vi "Main.vi"() -> ()   [LabVIEW 2021]
doc: "The myRIO Project template acquires acceleration data from the onboard accelerometer and displays the changes of acceleration values in a waveform chart."
uses:
  <vilib>/myRIO/Instrument Drivers/Onboard IO/I2C/typedefs/I2C User Configuration.ctl
  <vilib>/myRIO/Instrument Drivers/Onboard IO/I2C/typedefs/I2C Transfer Rate.ctl
  <vilib>/myRIO/Instrument Drivers/Onboard IO/DIO/typedefs/DIO Reference.ctl
  <vilib>/myRIO/Common/Instrument Driver Framework/Utilities/typedefs/myRIO Generic Hardware Reference.ctl
  <vilib>/myRIO/Common/Instrument Driver Framework/Utilities/typedefs/Hardware Version Enum.ctl
  <vilib>/myRIO/Common/Instrument Driver Framework/Utilities/typedefs/myRIO v1.0 Reference.ctl
  <vilib>/myRIO/Common/Instrument Driver Framework/Utilities/typedefs/Generic FPGA Reference.ctl
  <vilib>/myRIO/Common/Instrument Driver Framework/myRIO v1.0/DIO/typedefs/DIO Channels List.ctl
  <vilib>/myRIO/Common/Instrument Driver Framework/myRIO v1.0/DIO/typedefs/DIO Channels Enum.ctl
  <vilib>/userDefined/High Color/nirio_resource_hc.ctl
  <vilib>/myRIO/Instrument Drivers/Onboard IO/I2C/typedefs/I2C Reference.ctl
  <vilib>/myRIO/Common/Instrument Driver Framework/myRIO v1.0/I2C/typedefs/I2C Channels Enum.ctl
  <vilib>/myRIO/Instrument Drivers/Onboard IO/I2C/typedefs/I2C Configuration.ctl
  <vilib>/Platform/TimedLoop/XDataNode/timing_clust.ctl
  <vilib>/Platform/TimedLoop/XDataNode/nitl_modes.ctl
  <vilib>/Platform/TimedLoop/XDataNode/wakeup.ctl
  sketch_state.ctl
  <vilib>/myRIO/Instrument Drivers/Onboard IO/UART/typedef/VISA Configuration.ctl
  <vilib>/myRIO/Instrument Drivers/Onboard IO/SPI/typedefs/SPI User Configuration.ctl
  <vilib>/myRIO/Common/Instrument Driver Framework/myRIO v1.0/SPI/typedefs/SPI Clock Phase.ctl
  <vilib>/myRIO/Common/Instrument Driver Framework/myRIO v1.0/SPI/typedefs/SPI Clock Polarity.ctl
  <vilib>/myRIO/Common/Instrument Driver Framework/myRIO v1.0/SPI/typedefs/SPI Data Direction.ctl
  <vilib>/myRIO/Common/Instrument Driver Framework/myRIO v1.0/SPI/typedefs/SPI Frame Length.ctl
  <vilib>/myRIO/Instrument Drivers/Onboard IO/SPI/typedefs/SPI Reference.ctl
  <vilib>/myRIO/Common/Instrument Driver Framework/myRIO v1.0/SPI/typedefs/SPI Channels Enum.ctl
  <vilib>/myRIO/Instrument Drivers/Onboard IO/SPI/typedefs/SPI Configuration.ctl
  <vilib>/myRIO/Common/Instrument Driver Framework/myRIO v1.0/DIO/vis/myRIO v1.1 Open DIO.vi
  <vilib>/myRIO/Common/Instrument Driver Framework/myRIO v1.0/I2C/vis/myRIO v1.1 Open I2C.vi
  <vilib>/myRIO/Common/Instrument Driver Framework/Utilities/vis/Is FPGA Ref Available.vi
  <vilib>/myRIO/Common/Instrument Driver Framework/myRIO v1.0/SPI/vis/myRIO v1.1 Open SPI.vi
  <vilib>/myRIO/Common/Instrument Driver Framework/Utilities/vis/Validate Channels.vi
  <vilib>/myRIO/Common/Instrument Driver Framework/myRIO v1.0/DIO/vis/myRIO v1.0 Reserve DIO.vi
  <vilib>/myRIO/Common/Instrument Driver Framework/myRIO v1.0/I2C/vis/myRIO v1.0 Reserve I2C.vi
  <vilib>/myRIO/Common/Instrument Driver Framework/myRIO v1.0/SPI/vis/myRIO v1.0 Reserve SPI.vi
  <vilib>/myRIO/Common/Instrument Driver Framework/myRIO v1.0/DIO/vis/myRIO v1.0 Close DIO.vi
  <vilib>/myRIO/Common/Instrument Driver Framework/myRIO v1.0/Resource Manager/vis/myRIO v1.0 Reserve Channel List.vi
  <vilib>/myRIO/Common/Instrument Driver Framework/myRIO v1.0/DIO/vis/myRIO v1.0 Build MUX Configuration DIO.vi
  <vilib>/myRIO/Common/Instrument Driver Framework/myRIO v1.0/I2C/vis/myRIO v1.0 Build MUX Configuration I2C.vi
  <vilib>/myRIO/Common/Instrument Driver Framework/myRIO v1.0/SPI/vis/myRIO v1.0 Build MUX Configuration SPI.vi
  <vilib>/myRIO/Common/Instrument Driver Framework/myRIO v1.0/DIO/vis/myRIO v1.0 Unreserve DIO.vi
  <vilib>/myRIO/Common/Instrument Driver Framework/myRIO v1.0/Resource Manager/vis/myRIO v1.0 Reserve Channel.vi
  <vilib>/myRIO/Common/Instrument Driver Framework/myRIO v1.0/Resource Manager/vis/myRIO v1.0 Unreserve Channel.vi
  <vilib>/myRIO/Common/Instrument Driver Framework/myRIO v1.0/Resource Manager/vis/myRIO v1.0 Create Configuration List.vi
  <vilib>/myRIO/Common/Instrument Driver Framework/myRIO v1.0/Resource Manager/vis/myRIO v1.0 Unreserve Channel List.vi
  <vilib>/myRIO/Common/Instrument Driver Framework/myRIO v1.0/Resource Manager/vis/myRIO v1.0 Build Mutex Name.vi
  <vilib>/Utility/VariantDataType/GetNumericInfo.vi
  <vilib>/Utility/error.llb/Error Cluster From Error Code.vi
  <vilib>/myRIO/Common/Instrument Driver Framework/myRIO v1.0/myRIO v1.1 Open.vi
  <vilib>/myRIO/Common/Instrument Driver Framework/Utilities/vis/IO Manager.vi
  <vilib>/myRIO/Common/Instrument Driver Framework/Utilities/vis/Configuration Manager.vi
  <vilib>/myRIO/Common/Instrument Driver Framework/myRIO v1.0/Resource Manager/vis/myRIO v1.0 Configure IO.vi
  <vilib>/myRIO/Common/Instrument Driver Framework/myRIO v1.0/myRIO v1.0 Close.vi
  <vilib>/myRIO/Common/Instrument Driver Framework/myRIO v1.0/I2C/vis/myRIO v1.0 Configure I2C.vi
  <vilib>/myRIO/Common/Instrument Driver Framework/myRIO v1.0/I2C/vis/myRIO v1.0 Write I2C.vi
  <vilib>/Instr/_visa.llb/VISA Configure Serial Port (Instr).vi
  <vilib>/myRIO/Common/Instrument Driver Framework/myRIO v1.0/DIO/vis/myRIO v1.0 Write DIO.vi
  <vilib>/myRIO/Common/Instrument Driver Framework/myRIO v1.0/SPI/vis/myRIO v1.0 Configure SPI.vi
  <vilib>/myRIO/Common/Instrument Driver Framework/myRIO v1.0/SPI/vis/myRIO v1.0 Write Read SPI.vi
  <vilib>/myRIO/Common/Instrument Driver Framework/myRIO v1.0/DIO/vis/myRIO v1.0 Read DIO.vi
  <vilib>/myRIO/Common/Instrument Driver Framework/myRIO v1.0/I2C/vis/myRIO v1.0 Read I2C.vi
  <vilib>/myRIO/Common/Instrument Driver Framework/myRIO v1.0/DIO/vis/myRIO v1.0 Shutdown DIO.vi
  <vilib>/myRIO/Instrument Drivers/Onboard IO/DIO/vis/myRIO DIO Open.xnode
  <vilib>/myRIO/Instrument Drivers/Onboard IO/I2C/vis/myRIO I2C Open.xnode
  <vilib>/platform/TimedLoop/XDataNode/XDataNode.xnode
  <vilib>/myRIO/Express VI/Onboard IO/UART/UART Express VI.xnode
  <vilib>/myRIO/Express VI/Onboard IO/DO/DO Express VI.xnode
  <vilib>/myRIO/Express VI/Onboard IO/SPI/SPI Express VI.xnode
  <vilib>/myRIO/Instrument Drivers/Onboard IO/SPI/vis/myRIO SPI Open.xnode
  <vilib>/Platform/TimedLoop/XDataNode/XDNodeRunTimeDep.lvlib
  <vilib>/myRIO/Instrument Drivers/Onboard IO/DIO/DIO.lvlib
  <vilib>/myRIO/Instrument Drivers/Onboard IO/I2C/I2C.lvlib
  <vilib>/myRIO/Instrument Drivers/Onboard IO/SPI/SPI.lvlib
  <vilib>/myRIO/Instrument Drivers/Onboard IO/UART/UART.lvlib
panel:
  out "Bytes Read":u8[](array[numeric]) format="%x"
  out "X":i16
  out "Y":i16
  out "Z":i16
  in  "Stop Button":bool
  out "Waveform Chart":cluster{i16, i16, i16}(graph)
  out "INT_Source":bool[](array[boolean])
  out "Distance to Cabin":dbl
  out "Map":picture
  in  "Reset":bool
  in  "Left 2":bool
  in  "Forward":bool
  in  "Right 2":bool
  in  "Back":bool
  out "Light Detection":u8[](array[knob]) scale=0.0..255.0
  in  "Tree  Warning Dist (<)":u32
  out "Tree Warning":bool
  out "Ambient Temperature":dbl(slide) scale=0.0..40.0
  out "Alert":bool
  out "Ta":u8[](array[numeric])
  out "Thyst (hysteresis)":u8[](array[numeric]) format="%x"
  out "TSet":u8[](array[numeric]) format="%x"
  out "Sonic Distance (in)":u32
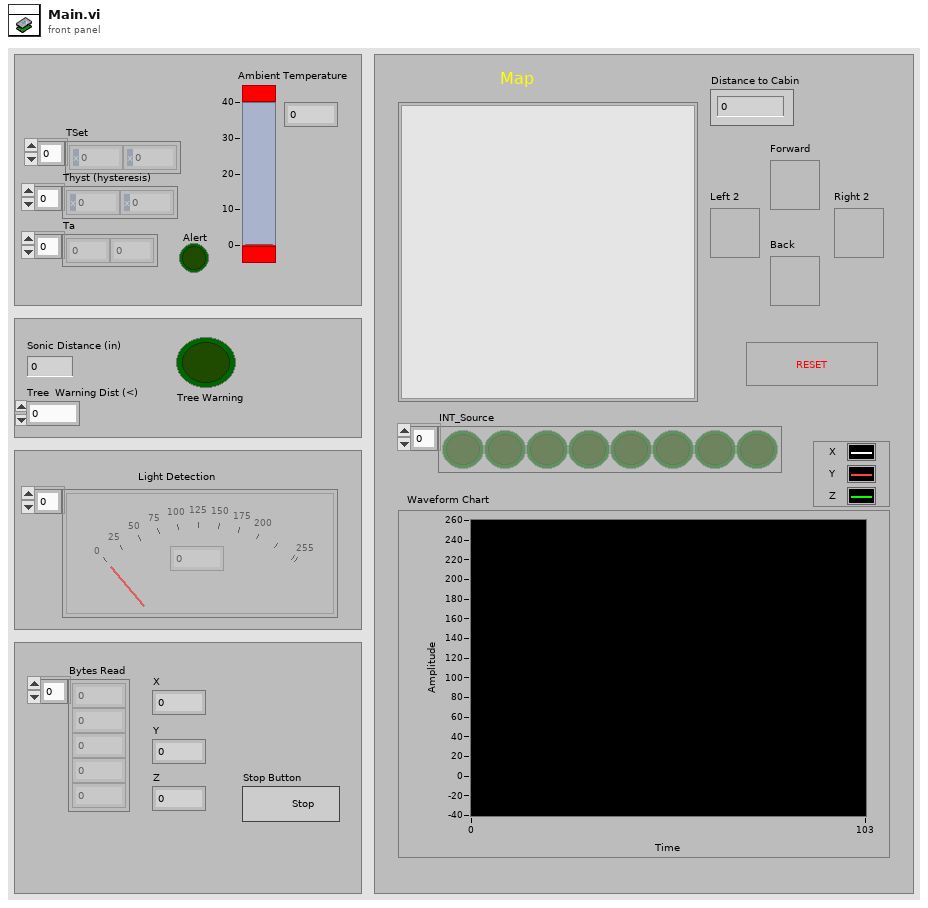
[diagram p1: front panel]
types:
  T1 = typedef "nirio_resource_hc.ctl" = tag
  T2 = typedef "Hardware Version Enum.ctl" = enum16{"Unknown", "myRIO-1900", "myRIO-1950", "roboRIO", "NI ELVIS RIO CM", "ELVIS III"}
  T3 = typedef "sketch_state.ctl" = enum16{"erase", "wait", "write"}
  T4 = typedef "UART.lvlib/VISA Configuration.ctl" = cluster{"baud rate (9600)":u32, "data bits (8)":u16, "parity (0:none)":enum16{"None", "Odd", "Even", "Mark", "Space"}, "stop bits (10: 1 bit)":u16, "flow control (0:none)":u16, "termination char\n(0xA = '\\n' = LF) ":u8, "Enable Termination\nChar (T)":bool, "timeout (10sec)":u32}
  T5 = typedef "DIO.lvlib/DIO Reference.ctl" = cluster{"myRIO Reference":T6, "DIO Channels List":T9}
  T6 = typedef "myRIO Generic Hardware Reference.ctl" = cluster{"myRIO Model":T2, "myRIO Hardware Reference":T7}
  T7 = typedef "myRIO v1.0 Reference.ctl" = cluster{"Generic FPGA Reference":T8, "Allow multiple opens":bool}
  T8 = typedef "Generic FPGA Reference.ctl" = refnum<k20>
  T9 = typedef "DIO Channels List.ctl" = T10[]
  T10 = typedef "DIO Channels Enum.ctl" = enum16{"Not Connected", "C/DIO0", "C/DIO1", "C/DIO2", "C/DIO3", "C/DIO4", "C/DIO5", "C/DIO6", "C/DIO7", "A/DIO0", "A/DIO1", "A/DIO2", "A/DIO3", "A/DIO4", "A/DIO5", "A/DIO6", "A/DIO7", "A/DIO8", "A/DIO9", "A/DIO10", "A/DIO11", "A/DIO12", "A/DIO13", "A/DIO14", "A/DIO15", "A/DIO16", "A/DIO17", "A/DIO18", "A/DIO19", "B/DIO0", "B/DIO1", "B/DIO2", "B/DIO3", "B/DIO4", "B/DIO5", "B/DIO6", "B/DIO7", "B/DIO8", "B/DIO9", "B/DIO10", "B/DIO11", "B/DIO12", "B/DIO13", "B/DIO14", "B/DIO15", "B/DIO16", "B/DIO17", "B/DIO18", "B/DIO19", "LED0", "LED1", "LED2", "LED3", "Button0", "DIO/DIO0", "DIO/DIO1", "DIO/DIO2", "DIO/DIO3", "DIO/DIO4", "DIO/DIO5", "DIO/DIO6", "DIO/DIO7", "DIO/DIO8", "DIO/DIO9", "SPI/CS0", "SPI/CS1", "SPI/CS2", "SPI/CS3", "LED RADIO (Green)", "LED RADIO (Red)", "LED COMM (Green)", "LED COMM (Red)", "LED MODE (Green)", "LED MODE (Red)"}
  T11 = typedef "SPI.lvlib/SPI Reference.ctl" = cluster{"myRIO Reference":T6, "SPI Channels Enum":T12, "SPI Configuration":T13}
  T12 = typedef "SPI Channels Enum.ctl" = enum16{"Not Connected", "A/SPI", "B/SPI", "SPI/SPI"}
  T13 = typedef "SPI.lvlib/SPI Configuration.ctl" = cluster{"Frequency [Hz]":dbl, "Clock Phase":T14, "Clock Polarity":T15, "Data Direction":T16, "Frame Length":T17}
  T14 = typedef "SPI Clock Phase.ctl" = enum8{"Leading", "Trailing"}
  T15 = typedef "SPI Clock Polarity.ctl" = enum8{"Low", "High"}
  T16 = typedef "SPI Data Direction.ctl" = enum8{"Most significant bit first", "Least significant bit first"}
  T17 = typedef "SPI Frame Length.ctl" = u8
  T18 = typedef "SPI.lvlib/SPI User Configuration.ctl" = cluster{"Frequency [Hz]":dbl, "Clock Phase":T14, "Clock Polarity":T15, "Data Direction":T16, "Frame Length":T17}
  T19 = typedef "XDNodeRunTimeDep.lvlib/timing_clust.ctl" = cluster{"Expected End [f-1]":u64, "Actual End [f-1]":u64, "Finished Late? [f-1]":bool, "Expected End [i-1]":u64, "Actual End [i-1]":u64, "Finished Late? [i-1]":bool, "Expected Start [i]":u64, "Actual Start [i]":u64, "Expected Start [f]":u64, "Actual Start [f]":u64, "Source Name":string, "Structure Name":string, "Period":i64, "Deadline":i64, "Offset":i64, "Start":i64, "Priority":i32, "Timeout":i32, "Mode":T20, "Wakeup Reason":T21, "Error":errorcluster, "Source Type":string, "Secondary Source Type":string, "Global End Time":u64, "Global Start Time":u64, "Frame Duration":u64, "Iteration Duration":u64, "Assigned CPU":i32, "I/O Scan Engine Mode":u32}
  T20 = typedef "XDNodeRunTimeDep.lvlib/nitl_modes.ctl" = enum32{"No Change", "Process missed periods, maintain original phase", "Discard missed periods, maintain original phase", "Process missed periods, ignore original phase", "Discard missed periods, ignore original phase"}
  T21 = typedef "XDNodeRunTimeDep.lvlib/wakeup.ctl" = enum32{"Normal", "Aborted", "Asynchronous wakeup", "Timing source error", "Timed loop error", "Timeout"}
  T22 = typedef "I2C.lvlib/I2C User Configuration.ctl" = cluster{"I2C Transfer Rate":T23}
  T23 = typedef "I2C.lvlib/I2C Transfer Rate.ctl" = enum16{"Standard mode (100 kbps)", "Fast mode (400 kbps)"}
  T24 = typedef "I2C.lvlib/I2C Reference.ctl" = cluster{"myRIO Reference":T6, "I2C Channels Enum":T25, "I2C Configuration":T26}
  T25 = typedef "I2C Channels Enum.ctl" = enum16{"Not Connected", "A/I2C", "B/I2C", "I2C/I2C"}
  T26 = typedef "I2C.lvlib/I2C Configuration.ctl" = cluster{"I2C Transfer Rate":T23}
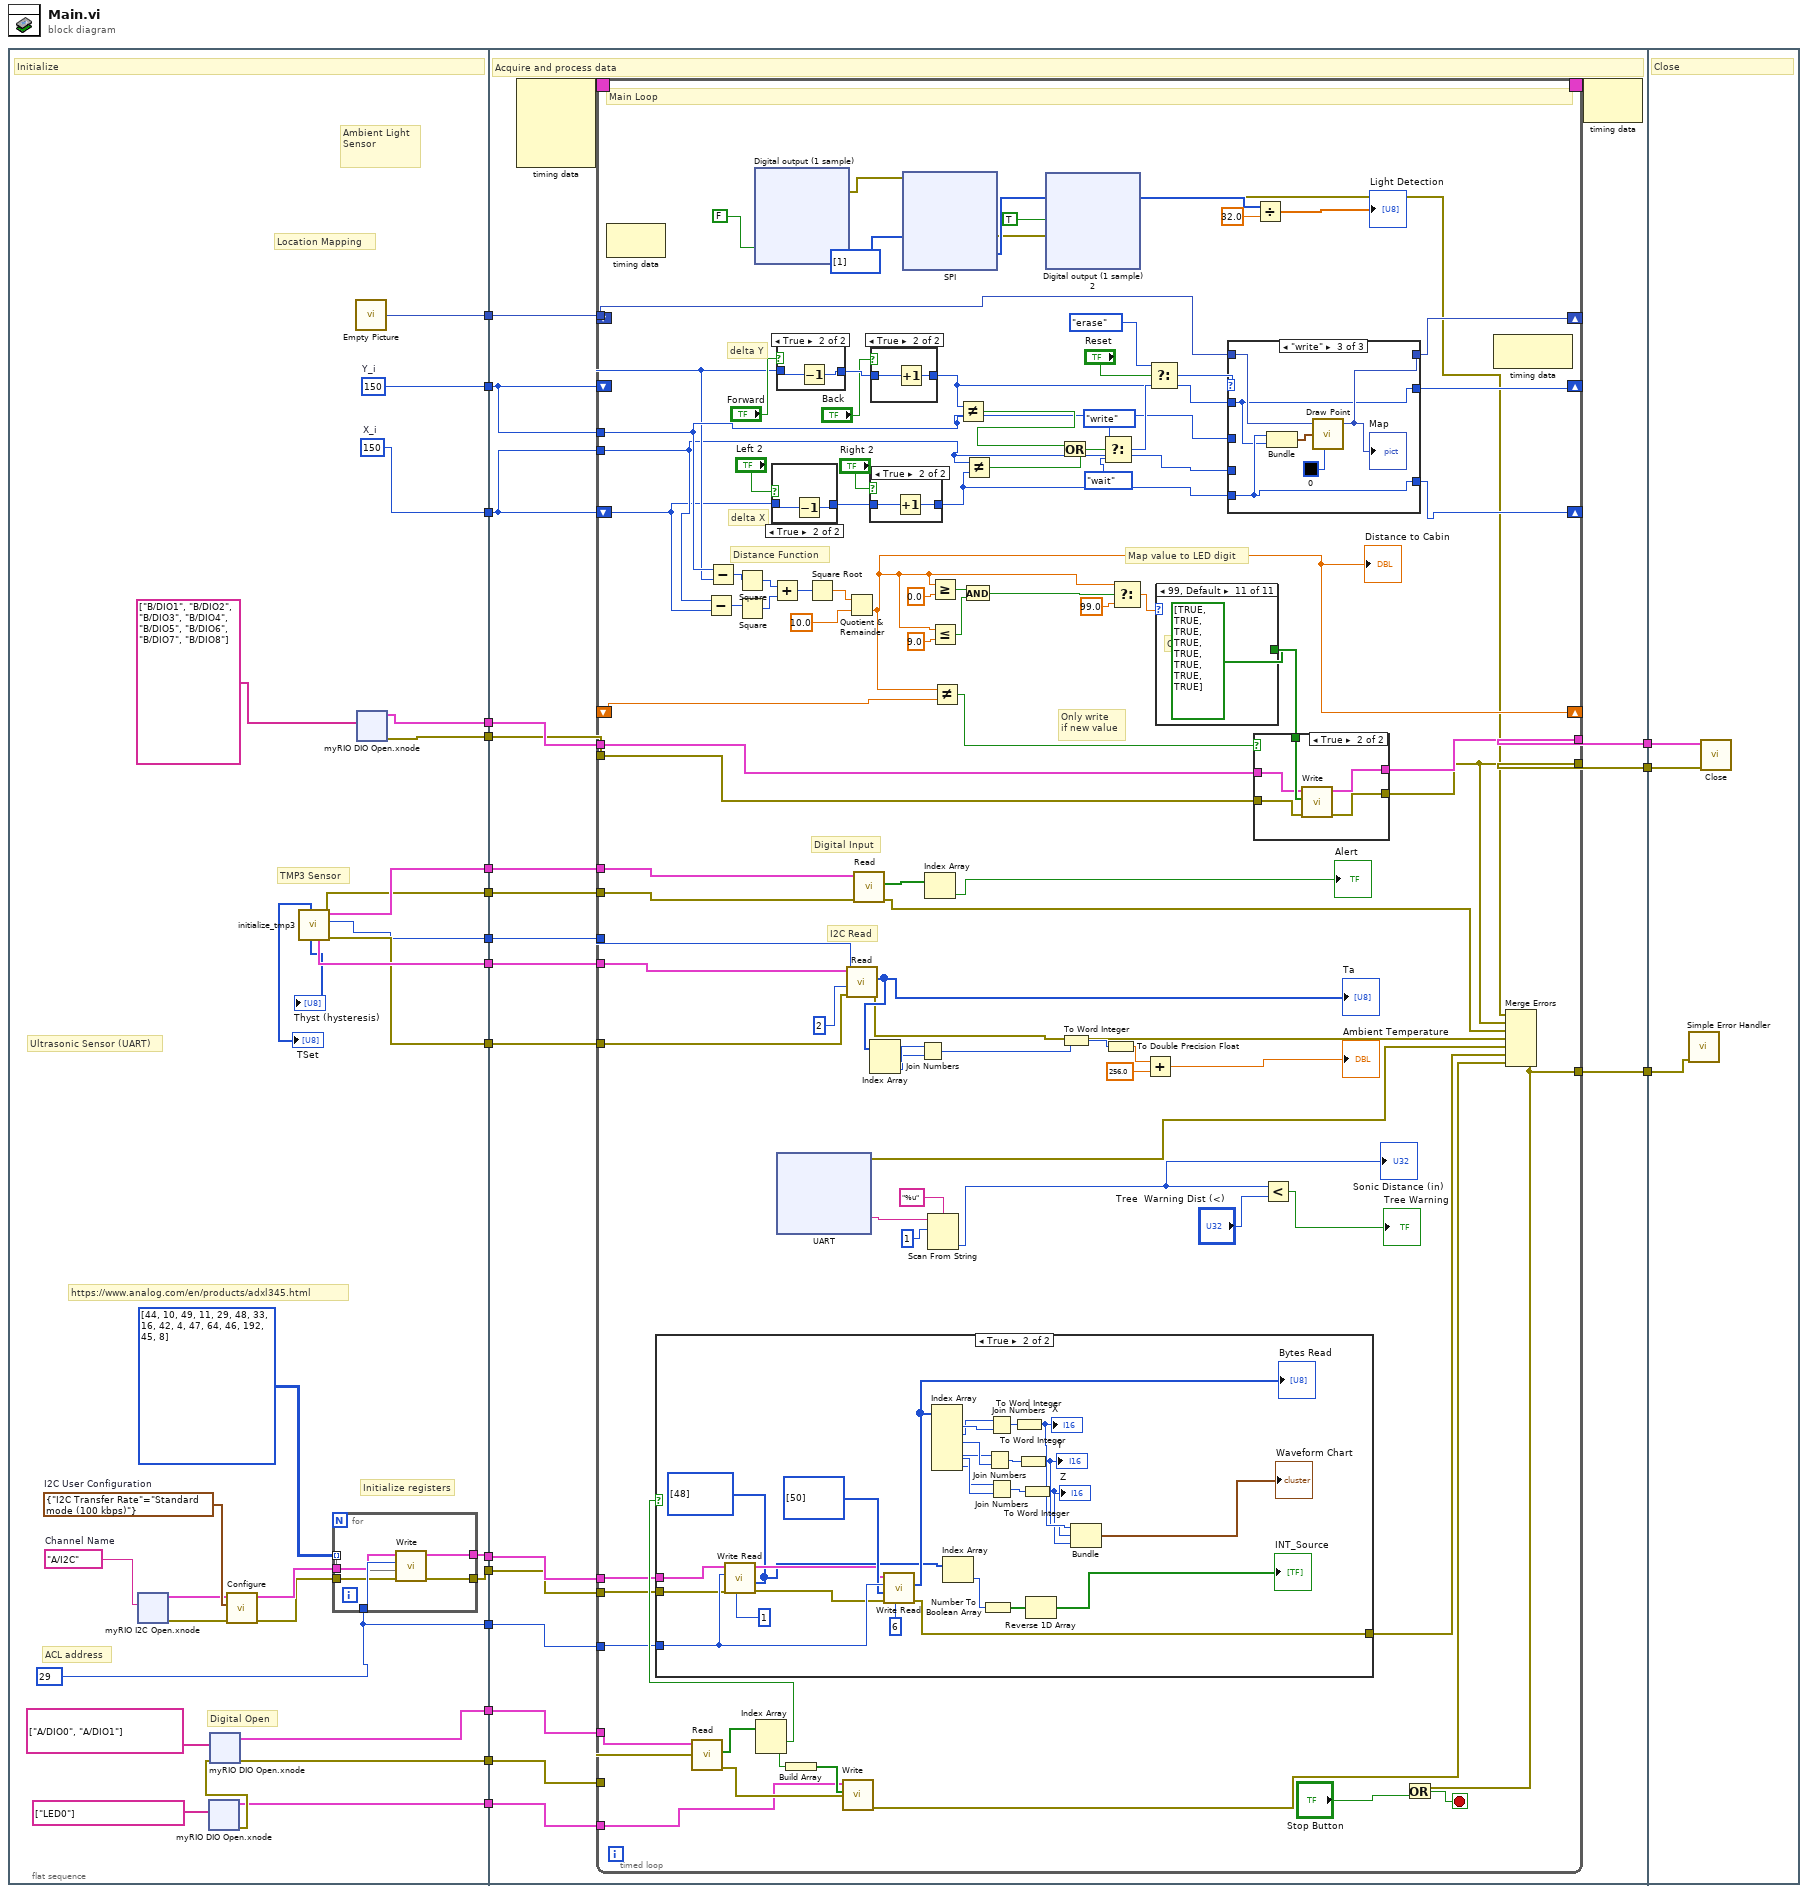
[diagram p0: block diagram]
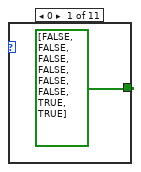
[diagram p4: hidden frame]
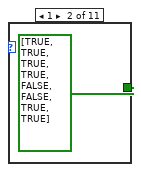
[diagram p5: hidden frame]
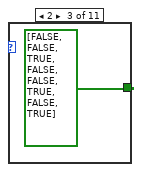
[diagram p6: hidden frame]
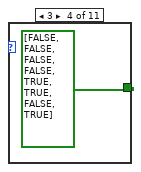
[diagram p7: hidden frame]
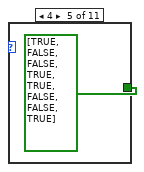
[diagram p8: hidden frame]
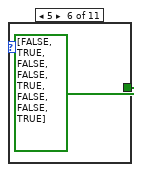
[diagram p9: hidden frame]
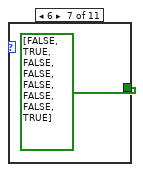
[diagram p10: hidden frame]
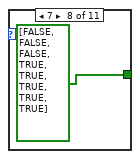
[diagram p11: hidden frame]
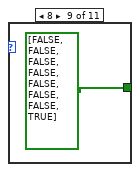
[diagram p12: hidden frame]
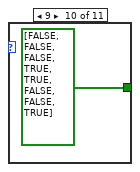
[diagram p13: hidden frame]
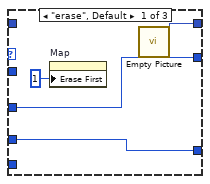
[diagram p14: hidden frame]
diagram:
  n1 = flat-sequence {
    tunnel: [w48] -> w19
    tunnel: [w47] -> w18
    tunnel: [w46] -> w17
    tunnel: [w45] -> w16
    tunnel: [w44] -> w15
    tunnel: [w43] -> w14
    tunnel: [w42] -> w13
    tunnel: [w41] -> w12
    tunnel: [w37] -> w11
    tunnel: [w36] -> w10
    tunnel: [w25] -> w9
    tunnel: [w24] -> w8
    tunnel: [w23] -> w7
    tunnel: [w22] -> w6
    tunnel: [w21] -> w5
    tunnel: [w20] -> w4
    tunnel: w19 -> [w137]
    tunnel: w18 -> [w136]
    tunnel: w17 -> [w135]
    tunnel: w16 -> [w134]
    tunnel: w15 -> [w133]
    tunnel: w14 -> [w132]
    tunnel: w13 -> [w131]
    tunnel: w12 -> [w130]
    tunnel: w11 -> [w129]
    tunnel: w10 -> [w128]
    tunnel: w9 -> [w127]
    tunnel: w8 -> [w126]
    tunnel: w7 -> [w125]
    tunnel: w6 -> [w124]
    tunnel: w5 -> [w123]
    tunnel: w4 -> [w122]
    tunnel: [w121] -> w3
    tunnel: [w120] -> w2
    tunnel: [w119] -> w1
    tunnel: w3 -> [w439]
    tunnel: w2 -> [w438]
    tunnel: w1 -> [w437]
    frame #0 {
      w23 = u8 29 ("Slave Address (7-bit)")
      w34 = T22 {"I2C Transfer Rate"=enum."Standard mode (100 kbps)"}  # I2C User Configuration
      w35 = tag "A/I2C"  # Channel Name
      w42 = 150  # Y_i
      w41 = 150  # X_i
      # "Digital Open"
      # "ACL address"
      # "https://www.analog.com/en/products/adxl345.html"
      # "Initialize registers"
      # "Ultrasonic Sensor (UART)"
      # "Ambient Light\nSensor"
      # "Location Mapping"
      # "TMP3 Sensor"
      # "Initialize"
      n2 = xnode "myRIO I2C Open.xnode"("Channel Name"=w35) -> ("error out"=w32:errorcluster, "I2C Ref Out"=w33:T24)  [unwired: 2 in]
      n3 = xnode "myRIO DIO Open.xnode"("Channel Names"=tag[] ["LED0"]) -> ("error out"=w26:errorcluster, "DIO Ref Out"=w20:T5)  [unwired: 2 in]
      n4 = xnode "myRIO DIO Open.xnode"("error in (no error)"=w26, "Channel Names"=tag[] ["A/DIO0", "A/DIO1"]) -> ("error out"=w21:errorcluster, "DIO Ref Out"=w22:T5)  [unwired: 1 in]
      n5 = call <vilib>:"Configure.vi"("error in (no error)"=w32, "I2C User Configuration"=w34, "I2C Ref In"=w33) -> ("error out"=w30:errorcluster, "I2C Ref Out"=w31:T24)  [unwired: 7 in]
      n6 = call "initialize_tmp3.vi"() -> (0:"error out"=w47:errorcluster, 1:"error out"=w45:errorcluster, "Slave Address (7-bit)"=w44:u8, "DIO Ref Out"=w46:T5, "I2C Ref Out"=w48:T24, "Thyst (hysteresis)"=→"Thyst (hysteresis)":u8[], "TSet"=→"TSet":u8[])  [unwired: 4 in, 1 out]
      n7 = for {
        tunnel: w23 -> [w86]
        tunnel: w31 -> [w85]
        tunnel: w30 -> [w84]
        tunnel: i32[][] [[44, 10], [49, 11], [29, 48], [33, 16], [42, 4], [47, 64], [46, 192], [45, 8]] -> [w83] mode=indexing
        tunnel: [w82] -> w25
        tunnel: [w81] -> w24
        n8 = call <vilib>:"Write.vi"("error in (no error)"=w84, "Bytes to Write"=w83, "Slave Address (7-bit)"=w86, "I2C Ref In"=w85) -> ("error out"=w81:errorcluster, "I2C Ref Out"=w82:T24)  [unwired: 6 in]
      }
      n9 = call "Empty Picture"() -> ("empty picture"=w43:picture)
      n10 = xnode ("myRIO DIO Open.xnode")("Channel Names"=tag[] ["B/DIO1", "B/DIO2", "B/DIO3", "B/DIO4", "B/DIO5", "B/DIO6", "B/DIO7", "B/DIO8"]) -> ("error out"=w36:errorcluster, "DIO Ref Out"=w37:T5)  [unwired: 2 in]
    }
    frame #1 {
      # "Acquire and process data"
      n11 = node-c288() -> (w139:T19)  [unwired: 4 in]
      n12 = timed-loop {
        timing: w139 -> [_]
        timing-out: [_] -> w138
        tunnel: w137 -> [w226]
        tunnel: w136 -> [w225]
        tunnel: w135 -> [w224]
        tunnel: w134 -> [w223]
        tunnel: w133 -> [w222]
        tunnel: w132 -> [w200]
        tunnel: w131 -> [w188]
        tunnel: w130 -> [w186]
        shift-right: [w199] -> _
        shift-left: _ -> [_]
        shift-right: [w198] -> _
        shift-left: w131 -> [w187]
        shift-right: [w197] -> _
        shift-left: w130 -> [w185]
        tunnel: w129 -> [w177]
        tunnel: w128 -> [w176]
        tunnel: [w175] -> w120
        tunnel: [w149] -> w121
        shift-right: [w173] -> _
        shift-left: _ -> [w174]
        tunnel: w127 -> [w166]
        tunnel: w126 -> [w165]
        tunnel: w125 -> [w164]
        tunnel: w124 -> [w163]
        tunnel: w123 -> [w162]
        tunnel: w122 -> [w161]
        tunnel: [w145] -> w119
        stop <- w146 stop-if-true
        # "Only write\nif new value"
        # "Map value to LED digit"
        # "Distance Function"
        # "delta X"
        # "delta Y"
        # "I2C Read"
        # "Digital Input"
        # "Main Loop"
        n13 = node-c288() -> ()  [unwired: 1 in, 1 out]
        n14 = call <vilib>:"Read.vi"("error in (no error)"=w162, "DIO Ref In"=w163) -> ("error out"=w171:errorcluster, "Values"=w170:bool[])  [unwired: 7 in, 1 out]
        n15 = Subtract(x=w186, y=w185) -> (x-y=w184:i32)
        n16 = Subtract(x=w188, y=w187) -> (x-y=w183:i32)
        n17 = Square(x=w183) -> (x^2=w182:i32)
        n18 = Square(x=w184) -> (x^2=w181:i32)
        n19 = xnode "Digital output (1 sample)"("A/DIO2 (Pin 15)"=FALSE) -> ("error out"=w158:errorcluster)  [unwired: 1 in]
        n20 = Index Array(array=w170) -> (element #1=w169:bool, element #2=w168:bool)  [unwired: 2 in]
        n21 = case shown="True" w169 {
          tunnel: w164 -> [_ w389]
          tunnel: w165 -> [w362 w365]
          tunnel: [w362 w364] -> w152
          tunnel: w166 -> [_ w363]
          frame False {
          }
          frame True {
            w369 = u8[] [48] ("Bytes to Write")
            n22 = call <vilib>:"Write Read.vi"("Byte Count"=u32 1, "error in (no error)"=w365, "Bytes to Write"=w369, "Slave Address (7-bit)"=w389, "I2C Ref In"=w363) -> ("error out"=w386:errorcluster, "I2C Ref Out"=w387:T24)  [unwired: 3 in, 1 out]
            n23 = call <vilib>:"Write Read.vi"("Byte Count"=u32 6, "error in (no error)"=w386, "Bytes to Write"=u8[] [50], "Slave Address (7-bit)"=w389, "I2C Ref In"=w387) -> ("error out"=w364:errorcluster, "Bytes Read"=w383:u8[])  [unwired: 3 in, 1 out]
            "Bytes Read" <- w383
            n24 = Index Array(array=w383) -> (element #1=w382:u8, element #2=w381:u8, element #3=w379:u8, element #4=w378:u8, element #5=w377:u8, element #6=w376:u8)  [unwired: 6 in]
            n25 = Index Array(array=w369) -> (element=w368:u8)  [unwired: 1 in]
            n26 = Number To Boolean Array(number=w368) -> (Boolean array=w367:bool[])
            n27 = Join Numbers(hi=w378, lo=w379) -> ((hi.lo)=w375:u16)
            n28 = Join Numbers(hi=w381, lo=w382) -> ((hi.lo)=w380:u16)
            n29 = Join Numbers(hi=w376, lo=w377) -> ((hi.lo)=w374:u16)
            n30 = To Word Integer(number=w380) -> (16bit integer=w373:i16)
            "X" <- w373
            n31 = To Word Integer(number=w375) -> (16bit integer=w372:i16)
            "Y" <- w372
            n32 = To Word Integer(number=w374) -> (16bit integer=w371:i16)
            "Z" <- w371
            n33 = Reverse 1D Array(array=w367) -> (reversed array=→"INT_Source":bool[])
            n34 = Bundle(w373, w372, w371) -> (→"Waveform Chart":cluster{i16, i16, i16})  [unwired: 1 in]
          }
        }
        n35 = case shown="True" "Left 2" {
          tunnel: [w427 w429] -> w212
          tunnel: w185 -> [w427 w428]
          frame False {
          }
          frame True {
            n36 = Decrement(x=w428) -> (x-1=w429:i32)
          }
        }
        n37 = Add(x=w182, y=w181) -> (x+y=w180:i32)
        n38 = case shown="True" "Forward" {
          tunnel: [w430 w432] -> w216
          tunnel: w187 -> [w430 w431]
          frame False {
          }
          frame True {
            n39 = Decrement(x=w431) -> (x-1=w432:i32)
          }
        }
        n40 = xnode "UART"() -> ("Characters Read"=w143:string, "error out"=w140:errorcluster)  [unwired: 1 in]
        n41 = Build Array(w168) -> (w167:bool[])
        n42 = Square Root(x=w180) -> (sqrt(x)=w179:dbl)
        n43 = call <vilib>:"Write.vi"("error in (no error)"=w171, "Values"=w167, "DIO Ref In"=w161) -> ("error out"=w153:errorcluster)  [unwired: 6 in, 1 out]
        n44 = Quotient & Remainder(x=w179, y=10.0) -> (floor(x/y)=w173:dbl)  [unwired: 1 out]
        "Distance to Cabin" <- w173
        n45 = call <vilib>:"Read.vi"("error in (no error)"=w225, "Byte Count"=u32 2, "Slave Address (7-bit)"=w222, "I2C Ref In"=w226) -> ("error out"=w151:errorcluster, "Bytes Read"=w233:u8[])  [unwired: 4 in, 1 out]
        "Ta" <- w233
        n46 = call <vilib>:"Read.vi"("error in (no error)"=w223, "DIO Ref In"=w224) -> ("error out"=w150:errorcluster, "Values"=w235:bool[])  [unwired: 7 in, 1 out]
        n47 = case shown="True" "Right 2" {
          tunnel: [w421 w423] -> w201
          tunnel: w212 -> [w421 w422]
          frame False {
          }
          frame True {
            n48 = Increment(x=w422) -> (x+1=w423:i32)
          }
        }
        n49 = Index Array(array=w233) -> (element #1=w232:u8, element #2=w231:u8)  [unwired: 2 in]
        n50 = case shown="True" "Back" {
          tunnel: [w424 w426] -> w202
          tunnel: w216 -> [w424 w425]
          frame False {
          }
          frame True {
            n51 = Increment(x=w425) -> (x+1=w426:i32)
          }
        }
        n52 = xnode "SPI"("Frames to Write"=u16[] [1], "error in (no error)"=w158) -> ("Frames Read"=w160:u16[], "error out"=w157:errorcluster)
        n53 = Join Numbers(hi=w232, lo=w231) -> ((hi.lo)=w230:u16)
        n54 = Index Array(array=w235) -> (element=→"Alert":bool)  [unwired: 1 in]
        n55 = Scan From String(format string="%u", input string=w143, initial scan location=u32 1) -> (output 1=w141:u32)  [unwired: 2 in, 3 out]
        "Sonic Distance (in)" <- w141
        n56 = Greater Or Equal?(x=w173, y=0.0) -> (x >= y?=w193:bool)
        n57 = Less Or Equal?(x=w173, y=9.0) -> (x <= y?=w191:bool)
        n58 = Not Equal?(x=w173, y=w174) -> (x != y?=w172:bool)
        n59 = Not Equal?(x=w202, y=w188) -> (x != y?=w209:bool)
        n60 = And(x=w193, y=w191) -> (x .and. y?=w190:bool)
        n61 = Not Equal?(x=w186, y=w201) -> (x != y?=w208:bool)
        n62 = xnode "Digital output (1 sample) 2"("A/DIO2 (Pin 15)"=TRUE ("A/DIO0 (Pin 11)"), "error in (no error)"=w157) -> ("error out"=w148:errorcluster)
        n63 = Or(x=w209, y=w208) -> (x .or. y?=w207:bool)
        n64 = To Word Integer(number=w230) -> (16bit integer=w229:i16)
        n65 = Select(t=sketch_state."write", s=w207, f=sketch_state."wait") -> (s? t:f=w204:T3)
        n66 = To Double Precision Float(number=w229) -> (double precision float=w228:dbl)
        n67 = Select(t=w173, s=w190, f=99.0) -> (s? t:f=w189:dbl)
        n68 = Add(x=w228, y=256.0) -> (x+y=→"Ambient Temperature":dbl)
        n69 = Select(t=sketch_state."erase", s="Reset", f=w204) -> (s? t:f=w203:T3)
        n70 = case shown="99, Default" w189 {
          tunnel: [bool[] [FALSE, FALSE, FALSE, FALSE, FALSE, FALSE, TRUE, TRUE] bool[] [TRUE, TRUE, TRUE, TRUE, FALSE, FALSE, TRUE, TRUE] bool[] [FALSE, FALSE, TRUE, FALSE, FALSE, TRUE, FALSE, TRUE] bool[] [FALSE, FALSE, FALSE, FALSE, TRUE, TRUE, FALSE, TRUE] bool[] [TRUE, FALSE, FALSE, TRUE, TRUE, FALSE, FALSE, TRUE] bool[] [FALSE, TRUE, FALSE, FALSE, TRUE, FALSE, FALSE, TRUE] bool[] [FALSE, TRUE, FALSE, FALSE, FALSE, FALSE, FALSE, TRUE] bool[] [FALSE, FALSE, FALSE, TRUE, TRUE, TRUE, TRUE, TRUE] bool[] [FALSE, FALSE, FALSE, FALSE, FALSE, FALSE, FALSE, TRUE] bool[] [FALSE, FALSE, FALSE, TRUE, TRUE, FALSE, FALSE, TRUE] bool[] [TRUE, TRUE, TRUE, TRUE, TRUE, TRUE, TRUE, TRUE]] -> w195
          frame 0 {
            # "0"
          }
          frame 1 {
            # "1"
          }
          frame 2 {
            # "2"
          }
          frame 3 {
            # "3"
          }
          frame 4 {
            # "4"
          }
          frame 5 {
            # "5"
          }
          frame 6 {
            # "6"
          }
          frame 7 {
            # "7"
          }
          frame 8 {
            # "8"
          }
          frame 9 {
            # "9"
          }
          frame 99, Default {
            # "Off."
          }
        }
        n71 = case shown="\"write\"" w203 {
          tunnel: w200 -> [_ w414 w418]
          tunnel: [w411 w414 w417] -> w199
          tunnel: w202 -> [_ w413 w415]
          tunnel: w188 -> [w410 _ _]
          tunnel: w186 -> [w409 _ _]
          tunnel: w201 -> [_ w412 w416]
          tunnel: [w410 w413 w415] -> w198
          tunnel: [w409 w412 w416] -> w197
          frame "erase", Default {
            n72 = property on="Map" class="Pict"("Erase First"=u8 1 ("Write Attribute")) -> ()  [unwired: 2 in, 2 out]
            n73 = call "Empty Picture"() -> ("empty picture"=w411:picture)
          }
          frame "wait" {
          }
          frame "write" {
            n74 = Bundle("X_i"=w416, "Y_i"=w415) -> (w419:cluster{"X_i":i32, "Y_i":i32})  [unwired: 1 in]
            n75 = call <vilib>:"Draw Point.vi"("picture"=w418, "point(x,y)"=w419, "color(black)"=u32 0 ("PEN COLOR")) -> ("new picture"=w417:picture)  [unwired: 6 in]
            "Map" <- w417
          }
        }
        n76 = case shown="True" w172 {
          tunnel: w195 -> [_ w396]
          tunnel: w177 -> [w390 w395]
          tunnel: w176 -> [w391 w394]
          tunnel: [w390 w393] -> w175
          tunnel: [w391 w392] -> w149
          frame False {
          }
          frame True {
            n77 = call <vilib>:"Write.vi"("error in (no error)"=w394, "Values"=w396, "DIO Ref In"=w395) -> ("error out"=w392:errorcluster, "DIO Ref Out"=w393:T5)  [unwired: 6 in]
          }
        }
        n78 = Divide(x=w160, y=32.0) -> (x/y=→"Light Detection":dbl[])
        n79 = Less?(x=w141, y="Tree  Warning Dist (<)") -> (x < y?=→"Tree Warning":bool)
        n80 = node-c288() -> ()  [unwired: 1 in, 1 out]
        n81 = Merge Errors(w148, w149, w150, w151, w140, w152, w153) -> (w145:errorcluster)
        n82 = Or(x=w145, y="Stop Button") -> (x .or. y?=w146:bool)
      }
      n83 = node-c288(w138) -> ()  [unwired: 1 out]
    }
    frame #2 {
      # "Close"
      n84 = call <vilib>:"Simple Error Handler.vi"("error in (no error)"=w437) -> ()  [unwired: 4 in, 5 out]
      n85 = call <vilib>:"Close.vi"("error in (no error)"=w439, "DIO Ref In"=w438) -> ()  [unwired: 9 in, 1 out]
    }
  }
